vi "rszvl Instrument Options.vi"(0 "VISA resource name":refnum<visa-resource-name>, 11 "error in (no error)":errorcluster) -> (4 "VISA resource name out":refnum<visa-resource-name>, 10 "Options List":string, 15 "error out":errorcluster)   [LabVIEW 2014]
doc: "This VI returns the instrument version number and the list of options which the instrument is equipped with.\n\nRemote-control command(s):\n*IDN?\n*OPT?"
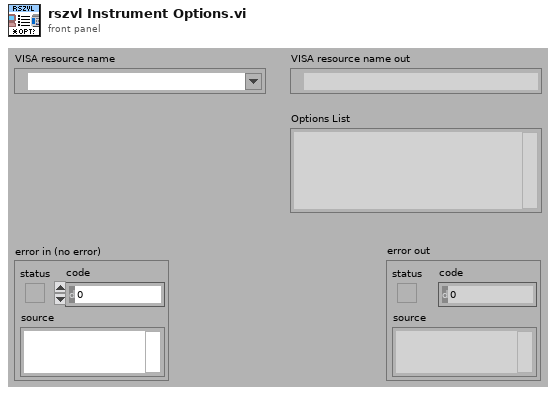
[diagram p1: front panel]
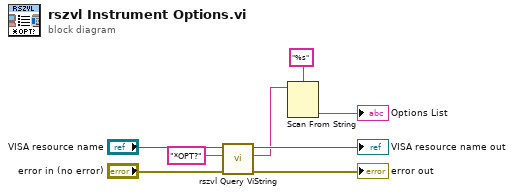
[diagram p0: block diagram]
diagram:
  n1 = call "rszvl Query ViString.vi"("error in (no error)"="error in (no error)", "Command"="*OPT?", "VISA resource name"="VISA resource name") -> ("error out"=→"error out":errorcluster, "Value"=w1:string, "VISA resource name out"=→"VISA resource name out":refnum<visa-resource-name>)  [unwired: 6 in]
  n2 = Scan From String(format string="%s", input string=w1) -> (output 1=→"Options List":string)  [unwired: 3 in, 3 out]
